vi "PDLM_GetDeviceData.vi"(8 "error in (no error)":errorcluster, 11 "USBIdx":i32) -> (0 "error out":errorcluster, 2 "Data":T1, 3 "return type":i32)   [LabVIEW 2017]
uses:
  PDLM_DeviceData.ctl
  PDLM_VersNum.ctl
  PDLM_DllPath_global.vi
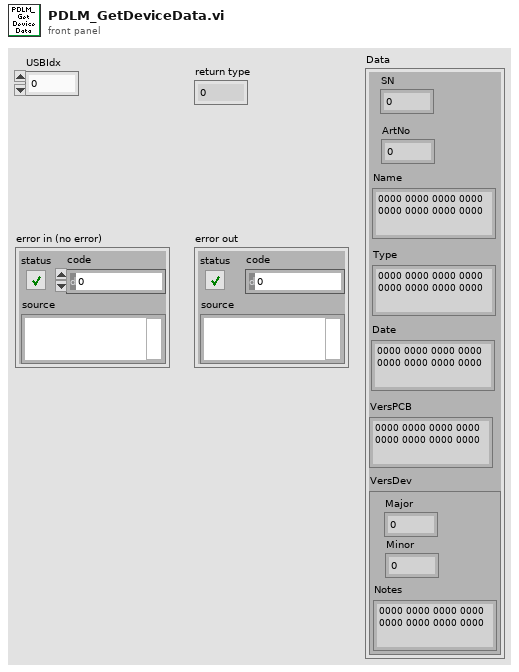
[diagram p1: front panel]
types:
  T1 = typedef "PDLM_DeviceData.ctl" = cluster{"SN":u32, "ArtNo":u32, "Name":string, "Type":string, "Date":string, "VersPCB":string, "VersDev":T2}
  T2 = typedef "PDLM_VersNum.ctl" = cluster{"Major":u16, "Minor":u16, "Notes":string}
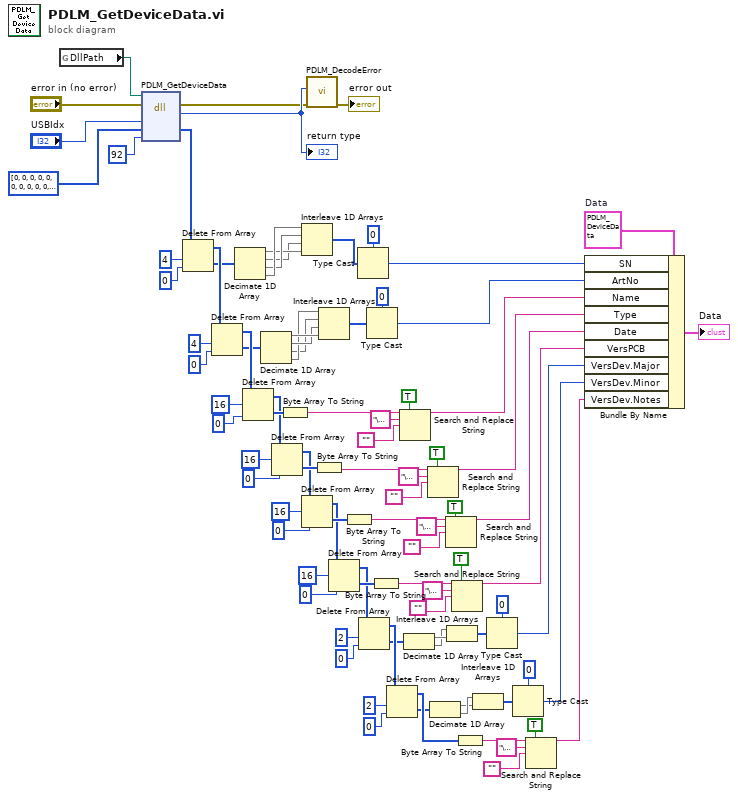
[diagram p0: block diagram]
diagram:
  w69 = T1 {"SN"=0, "ArtNo"=0, "Name"="\u0000\u0000\u0000\u0000\u0000\u0000\u0000\u0000\u0000\u0000\u0000\u0000\u0000\u0000\u0000\u0000", "Type"="\u0000\u0000\u0000\u0000\u0000\u0000\u0000\u0000\u0000\u0000\u0000\u0000\u0000\u0000\u0000\u0000", "Date"="\u0000\u0000\u0000\u0000\u0000\u0000\u0000\u0000\u0000\u0000\u0000\u0000\u0000\u0000\u0000\u0000", "VersPCB"="\u0000\u0000\u0000\u0000\u0000\u0000\u0000\u0000\u0000\u0000\u0000\u0000\u0000\u0000\u0000\u0000", "VersDev"={"Major"=0, "Minor"=0, "Notes"="\u0000\u0000\u0000\u0000\u0000\u0000\u0000\u0000\u0000\u0000\u0000\u0000\u0000\u0000\u0000\u0000"}}  # Data
  n1 = global read "PDLM_DllPath_global.vi" "DllPath"() -> (w88:path)
  n2 = dll-call lib="M:/_dev/progs/LabVIEW/_lib/PQ/Taiko/pdlm_lib.dll" fn="PDLM_GetDeviceData"(path in=w88, error in="error in (no error)", "USBIdx"="USBIdx", "Data"=u8[] [0, 0, 0, 0, 0, 0, 0, 0, 0, 0, 0, 0, 0, 0, 0, 0, 0, 0, 0, 0, 0, 0, 0, 0, 0, 0, 0, 0, 0, 0, 0, 0, 0, 0, 0, 0, 0, 0, 0, 0, 0, 0, 0, 0, 0, 0, 0, 0, 0, 0, 0, 0, 0, 0, 0, 0, 0, 0, 0, 0, 0, 0, 0, 0, 0, 0, 0, 0, 0, 0, 0, 0, 0, 0, 0, 0, 0, 0, 0, 0, 0, 0, 0, 0, 0, 0, 0, 0, 0, 0, 0, 0], "size"=u32 92) -> (error out=w90:errorcluster, "return type"=w91:i32, "Data"=w85:u8[])  [unwired: 3 in, 1 out]
  "return type" <- w91
  n3 = Delete From Array(array=w85, length=4, index=0) -> (deleted portion=w45:u8[], array with subset deleted=w79:u8[])
  n4 = Delete From Array(array=w79, length=4, index=0) -> (deleted portion=w39:u8[], array with subset deleted=w77:u8[])
  n5 = Decimate 1D Array(w45) -> (w41:u8[], w40:u8[], w42:u8[], w43:u8[])
  n6 = Delete From Array(array=w77, length=16, index=0) -> (deleted portion=w74:u8[], array with subset deleted=w70:u8[])
  n7 = Decimate 1D Array(w39) -> (w38:u8[], w37:u8[], w35:u8[], w36:u8[])
  n8 = Delete From Array(array=w70, length=16, index=0) -> (deleted portion=w73:u8[], array with subset deleted=w63:u8[])
  n9 = Byte Array To String(unsigned byte array=w74) -> (string=w25:string)
  n10 = Interleave 1D Arrays(w43, w42, w40, w41) -> (w44:u8[])
  n11 = Delete From Array(array=w63, length=16, index=0) -> (deleted portion=w64:u8[], array with subset deleted=w59:u8[])
  n12 = call "PDLM_DecodeError.vi"("error in (no error)"=w90, "code"=w91) -> ("error out"=→"error out":errorcluster)  [unwired: 7 in, 2 out]
  n13 = Byte Array To String(unsigned byte array=w73) -> (string=w17:string)
  n14 = Interleave 1D Arrays(w36, w35, w37, w38) -> (w34:u8[])
  n15 = Delete From Array(array=w59, length=16, index=0) -> (deleted portion=w62:u8[], array with subset deleted=w55:u8[])
  n16 = Byte Array To String(unsigned byte array=w64) -> (string=w12:string)
  n17 = Type Cast(type=u32 0, x=w44) -> (*(type *) &x=w68:u32)
  n18 = Delete From Array(array=w55, length=2, index=0) -> (deleted portion=w33:u8[], array with subset deleted=w48:u8[])
  n19 = Type Cast(type=u32 0, x=w34) -> (*(type *) &x=w67:u32)
  n20 = Byte Array To String(unsigned byte array=w62) -> (string=w7:string)
  n21 = Delete From Array(array=w48, length=2, index=0) -> (deleted portion=w27:u8[], array with subset deleted=w46:u8[])
  n22 = Search and Replace String(replace all?=TRUE ("replace all? (F)"), input string=w25, search string="\u0000", replace string="") -> (result string=w24:string)  [unwired: 4 in, 3 out]
  n23 = Decimate 1D Array(w33) -> (w32:u8[], w31:u8[])
  n24 = Search and Replace String(replace all?=TRUE ("replace all? (F)"), input string=w17, search string="\u0000", replace string="") -> (result string=w16:string)  [unwired: 4 in, 3 out]
  n25 = Decimate 1D Array(w27) -> (w28:u8[], w29:u8[])
  n26 = Search and Replace String(replace all?=TRUE ("replace all? (F)"), input string=w12, search string="\u0000", replace string="") -> (result string=w11:string)  [unwired: 4 in, 3 out]
  n27 = Interleave 1D Arrays(w31, w32) -> (w30:u8[])
  n28 = Search and Replace String(replace all?=TRUE ("replace all? (F)"), input string=w7, search string="\u0000", replace string="") -> (result string=w6:string)  [unwired: 4 in, 3 out]
  n29 = Byte Array To String(unsigned byte array=w46) -> (string=w2:string)
  n30 = Interleave 1D Arrays(w29, w28) -> (w26:u8[])
  n31 = Type Cast(type=u16 0, x=w30) -> (*(type *) &x=w52:u16)
  n32 = Type Cast(type=u16 0, x=w26) -> (*(type *) &x=w47:u16)
  n33 = Search and Replace String(replace all?=TRUE ("replace all? (F)"), input string=w2, search string="\u0000", replace string="") -> (result string=w1:string)  [unwired: 4 in, 3 out]
  n34 = Bundle By Name(cluster=w69, "SN"=w68, "ArtNo"=w67, "Name"=w24, "Type"=w16, "Date"=w11, "VersPCB"=w6, "VersDev.Major"=w52, "VersDev.Minor"=w47, "VersDev.Notes"=w1) -> (→"Data":T1)
